vi "Format CSV.vi"(8 "error in (no error)":errorcluster, 9 "delimiter":string=",", 10 "CSV File Input":path, 11 "Original CSV Format":enum16{"Format A", "Format B"}(ring)) -> (0 "error out":errorcluster, 1 "Parcel Length":i32[](array[numeric]), 2 "All Terminal Data":T1(array[cluster]))   [LabVIEW 2017] (continued)
  in  "Start Time Selection":u16(ring) items=["20:35.0", "20:35.0", "20:35.1", "20:35.1", "20:35.1", "20:35.2", "20:35.2", "20:35.2", "20:35.3", "20:35.3", "20:35.3", "20:35.4", "20:35.4", "20:35.4", "20:35.5", "20:35.5", "20:35.5", "20:35.6", "20:35.6", "20:35.6", "20:35.7", "20:35.7", "20:35.7", "20:35.8", "20:35.8", "20:35.8", "20:35.9", "20:35.9", "20:35.9", "20:36.0", "20:36.0", "20:36.0", "20:36.1", "20:36.1", "20:36.1", "20:36.2", "20:36.2", "20:36.2", "20:36.3", "20:36.3", "20:36.3", "20:36.4", "20:36.4", "20:36.4", "20:36.5", "20:36.5", "20:36.5", "20:36.6", "20:36.6", "20:36.6", "20:36.7", "20:36.7", "20:36.7", "20:36.8", "20:36.8", "20:36.8", "20:36.9", "20:36.9", "20:36.9", "20:37.0", "20:37.0", "20:37.0", "20:37.1", "20:37.1", "20:37.1", "20:37.2", "20:37.2", "20:37.2", "20:37.3", "20:37.3", "20:37.3", "20:37.4", "20:37.4", "20:37.4", "20:37.5", "20:37.5", "20:37.5", "20:37.6", "20:37.6", "20:37.6", "20:37.7", "20:37.7", "20:37.7", "20:37.8", "20:37.8", "20:37.8", "20:37.9", "20:37.9", "20:37.9", "20:38.0", "20:38.0", "20:38.0", "20:38.1", "20:38.1", "20:38.1", "20:38.2", "20:38.2", "20:38.2", "20:38.3", "20:38.3", "20:38.3", "20:38.4", "20:38.4", "20:38.4", "20:38.5", "20:38.5", "20:38.5", "20:38.6", "20:38.6", "20:38.6", "20:38.7", "20:38.7", "20:38.7", "20:38.8", "20:38.8", "20:38.8", "20:38.9", "20:38.9", "20:38.9", "20:39.0", "20:39.0", "20:39.0", "20:39.1", "20:39.1", "20:39.1", "20:39.2", "20:39.2", "20:39.2", "20:39.3", "20:39.3", "20:39.3", "20:39.4", "20:39.4", "20:39.4", "20:39.5", "20:39.5", "20:39.5", "20:39.6", "20:39.6", "20:39.6", "20:39.7", "20:39.7", "20:39.7", "20:39.8", "20:39.8", "20:39.8", "20:39.9", "20:39.9", "20:39.9", "20:40.0", "20:40.0", "20:40.0", "20:40.1", "20:40.1", "20:40.1", "20:40.2", "20:40.2", "20:40.2", "20:40.3", "20:40.3", "20:40.3", "20:40.4", "20:40.4", "20:40.4", "20:40.5", "20:40.5", "20:40.5", "20:40.6", "20:40.6", "20:40.6", "20:40.7", "20:40.7", "20:40.7", "20:40.8", "20:40.8", "20:40.8", "20:40.9", "20:40.9", "20:40.9", "20:41.0", "20:41.0", "20:41.0", "20:41.1", "20:41.1", "20:41.1", "20:41.2", "20:41.2", "20:41.2", "20:41.3", "20:41.3", "20:41.3", "20:41.4", "20:41.4", "20:41.4", "20:41.5", "20:41.5", "20:41.5", "20:41.6", "20:41.6", "20:41.6", "20:41.7", "20:41.7", "20:41.7", "20:41.8", "20:41.8", "20:41.8", "20:41.9", "20:41.9", "20:41.9", "20:42.0", "20:42.0", "20:42.0", "20:42.1", "20:42.1", "20:42.1", "20:42.2", "20:42.2", "20:42.2", "20:42.3", "20:42.3", "20:42.3", "20:42.4", "20:42.4", "20:42.4", "20:42.5", "20:42.5", "20:42.5", "20:42.6", "20:42.6", "20:42.6", "20:42.7", "20:42.7", "20:42.7", "20:42.8", "20:42.8", "20:42.8", "20:42.9", "20:42.9", "20:42.9", "20:43.0", "20:43.0", "20:43.0", "20:43.1", "20:43.1", "20:43.1", "20:43.2", "20:43.2", "20:43.2", "20:43.3", "20:43.3", "20:43.3", "20:43.4", "20:43.4", "20:43.4", "20:43.5", "20:43.5", "20:43.5", "20:43.6", "20:43.6", "20:43.6", "20:43.7", "20:43.7", "20:43.7", "20:43.8", "20:43.8", "20:43.8", "20:43.9", "20:43.9", "20:43.9", "20:44.0", "20:44.0", "20:44.0", "20:44.1", "20:44.1", "20:44.1", "20:44.2", "20:44.2", "20:44.2", "20:44.3", "20:44.3", "20:44.3", "20:44.4", "20:44.4", "20:44.4", "20:44.5", "20:44.5", "20:44.5", "20:44.6", "20:44.6", "20:44.6", "20:44.7", "20:44.7", "20:44.7", "20:44.8", "20:44.8", "20:44.8", "20:44.9", "20:44.9", "20:44.9", "20:45.0", "20:45.0", "20:45.0", "20:45.1", "20:45.1", "20:45.1", "20:45.2", "20:45.2", "20:45.2", "20:45.3", "20:45.3", "20:45.3", "20:45.4", "20:45.4", "20:45.4", "20:45.5", "20:45.5", "20:45.5", "20:45.6", "20:45.6", "20:45.6", "20:45.7", "20:45.7", "20:45.7", "20:45.8", "20:45.8", "20:45.8", "20:45.9", "20:45.9", "20:45.9", "20:46.0", "20:46.0", "20:46.0", "20:46.1", "20:46.1", "20:46.1", "20:46.2", "20:46.2", "20:46.2", "20:46.3", "20:46.3", "20:46.3", "20:46.4", "20:46.4", "20:46.4", "20:46.5", "20:46.5", "20:46.5", "20:46.6", "20:46.6", "20:46.6", "20:46.7", "20:46.7", "20:46.7", "20:46.8", "20:46.8", "20:46.8", "20:46.9", "20:46.9", "20:46.9", "20:47.0", "20:47.0", "20:47.0", "20:47.1", "20:47.1", "20:47.1", "20:47.2", "20:47.2", "20:47.2", "20:47.3", "20:47.3", "20:47.3", "20:47.4", "20:47.4", "20:47.4", "20:47.5", "20:47.5", "20:47.5", "20:47.6", "20:47.6", "20:47.6", "20:47.7", "20:47.7", "20:47.7", "20:47.8", "20:47.8", "20:47.8", "20:47.9", "20:47.9", "20:47.9", "20:48.0", "20:48.0", "20:48.0", "20:48.1", "20:48.1", "20:48.1", "20:48.2", "20:48.2", "20:48.2", "20:48.3", "20:48.3", "20:48.3", "20:48.4", "20:48.4", "20:48.4", "20:48.5", "20:48.5", "20:48.5", "20:48.6", "20:48.6", "20:48.6", "20:48.7", "20:48.7", "20:48.7", "20:48.8", "20:48.8", "20:48.8", "20:48.9", "20:48.9", "20:48.9", "20:49.0", "20:49.0", "20:49.0", "20:49.1", "20:49.1", "20:49.1", "20:49.2", "20:49.2", "20:49.2", "20:49.3", "20:49.3", "20:49.3", "20:49.4", "20:49.4", "20:49.4", "20:49.5", "20:49.5", "20:49.5", "20:49.6", "20:49.6", "20:49.6", "20:49.7", "20:49.7", "20:49.7", "20:49.8", "20:49.8", "20:49.8", "20:49.9", "20:49.9", "20:49.9", "20:50.0", "20:50.0", "20:50.0", "20:50.1", "20:50.1", "20:50.1", "20:50.2", "20:50.2", "20:50.2", "20:50.3", "20:50.3", "20:50.3", "20:50.4", "20:50.4", "20:50.4", "20:50.5", "20:50.5", "20:50.5", "20:50.6", "20:50.6", "20:50.6", "20:50.7", "20:50.7", "20:50.7", "20:50.8", "20:50.8", "20:50.8", "20:50.9", "20:50.9", "20:50.9", "20:51.0", "20:51.0", "20:51.0", "20:51.1", "20:51.1", "20:51.1", "20:51.2", "20:51.2", "20:51.2", "20:51.3", "20:51.3", "20:51.3", "20:51.4", "20:51.4", "20:51.4", "20:51.5", "20:51.5", "20:51.5", "20:51.6", "20:51.6", "20:51.6", "20:51.7", "20:51.7", "20:51.7", "20:51.8", "20:51.8", "20:51.8", "20:51.9", "20:51.9", "20:51.9", "20:52.0", "20:52.0", "20:52.0", "20:52.1", "20:52.1", "20:52.1", "20:52.2", "20:52.2", "20:52.2", "20:52.3", "20:52.3", "20:52.3", "20:52.4", "20:52.4", "20:52.4", "20:52.5", "20:52.5", "20:52.5", "20:52.6", "20:52.6", "20:52.6", "20:52.7", "20:52.7", "20:52.7", "20:52.8", "20:52.8", "20:52.8", "20:52.9", "20:52.9", "20:52.9", "20:53.0", "20:53.0", "20:53.0", "20:53.1", "20:53.1", "20:53.1", "20:53.2", "20:53.2", "20:53.2", "20:53.3", "20:53.3", "20:53.3", "20:53.4", "20:53.4", "20:53.4", "20:53.5", "20:53.5", "20:53.5", "20:53.6", "20:53.6", "20:53.6", "20:53.7", "20:53.7", "20:53.7", "20:53.8", "20:53.8", "20:53.8", "20:53.9", "20:53.9", "20:53.9", "20:54.0", "20:54.0", "20:54.0", "20:54.1", "20:54.1", "20:54.1", "20:54.2", "20:54.2", "20:54.2", "20:54.3", "20:54.3", "20:54.3", "20:54.4", "20:54.4", "20:54.4", "20:54.5", "20:54.5", "20:54.5", "20:54.6", "20:54.6", "20:54.6", "20:54.7", "20:54.7", "20:54.7", "20:54.8", "20:54.8", "20:54.8", "20:54.9", "20:54.9", "20:54.9", "20:55.0", "20:55.0", "20:55.0", "20:55.1", "20:55.1", "20:55.1", "20:55.2", "20:55.2", "20:55.2", "20:55.3", "20:55.3", "20:55.3", "20:55.4", "20:55.4", "20:55.4", "20:55.5", "20:55.5", "20:55.5", "20:55.6", "20:55.6", "20:55.6", "20:55.7", "20:55.7", "20:55.7", "20:55.8", "20:55.8", "20:55.8", "20:55.9", "20:55.9", "20:55.9", "20:56.0", "20:56.0", "20:56.0", "20:56.1", "20:56.1", "20:56.1", "20:56.2", "20:56.2", "20:56.2", "20:56.3", "20:56.3", "20:56.3", "20:56.4", "20:56.4", "20:56.4", "20:56.5", "20:56.5", "20:56.5", "20:56.6", "20:56.6", "20:56.6", "20:56.7", "20:56.7", "20:56.7", "20:56.8", "20:56.8", "20:56.8", "20:56.9", "20:56.9", "20:56.9", "20:57.0", "20:57.0", "20:57.0", "20:57.1", "20:57.1", "20:57.1", "20:57.2", "20:57.2", "20:57.2", "20:57.3", "20:57.3", "20:57.3", "20:57.4", "20:57.4", "20:57.4", "20:57.5", "20:57.5", "20:57.5", "20:57.6", "20:57.6", "20:57.6", "20:57.7", "20:57.7", "20:57.7", "20:57.8", "20:57.8", "20:57.8", "20:57.9", "20:57.9", "20:57.9", "20:58.0", "20:58.0", "20:58.0", "20:58.1", "20:58.1", "20:58.1", "20:58.2", "20:58.2", "20:58.2", "20:58.3", "20:58.3", "20:58.3", "20:58.4", "20:58.4", "20:58.4", "20:58.5", "20:58.5", "20:58.5", "20:58.6", "20:58.6", "20:58.6", "20:58.7", "20:58.7", "20:58.7", "20:58.8", "20:58.8", "20:58.8", "20:58.9", "20:58.9", "20:58.9", "20:59.0", "20:59.0", "20:59.0", "20:59.1", "20:59.1", "20:59.1", "20:59.2", "20:59.2", "20:59.2", "20:59.3", "20:59.3", "20:59.3", "20:59.4", "20:59.4", "20:59.4", "20:59.5", "20:59.5", "20:59.5", "20:59.6", "20:59.6", "20:59.6", "20:59.7", "20:59.7", "20:59.7", "20:59.8", "20:59.8", "20:59.8", "20:59.9", "20:59.9", "20:59.9", "21:00.0", "21:00.0", "21:00.0", "21:00.1", "21:00.1", "21:00.1", "21:00.2", "21:00.2", "21:00.2", "21:00.3", "21:00.3", "21:00.3", "21:00.4", "21:00.4", "21:00.4", "21:00.5", "21:00.5", "21:00.5", "21:00.6", "21:00.6", "21:00.6", "21:00.7", "21:00.7", "21:00.7", "21:00.8", "21:00.8", "21:00.8", "21:00.9", "21:00.9", "21:00.9", "21:01.0", "21:01.0", "21:01.0", "21:01.1", "21:01.1", "21:01.1", "21:01.2", "21:01.2", "21:01.2", "21:01.3", "21:01.3", "21:01.3", "21:01.4", "21:01.4", "21:01.4", "21:01.5", "21:01.5", "21:01.5", "21:01.6", "21:01.6", "21:01.6", "21:01.7", "21:01.7", "21:01.7", "21:01.8", "21:01.8", "21:01.8", "21:01.9", "21:01.9", "21:01.9", "21:02.0", "21:02.0", "21:02.0", "21:02.1", "21:02.1", "21:02.1", "21:02.2", "21:02.2", "21:02.2", "21:02.3", "21:02.3", "21:02.3", "21:02.4", "21:02.4", "21:02.4", "21:02.5", "21:02.5", "21:02.5", "21:02.6", "21:02.6", "21:02.6", "21:02.7", "21:02.7", "21:02.7", "21:02.8", "21:02.8", "21:02.8", "21:02.9", "21:02.9", "21:02.9", "21:03.0", "21:03.0", "21:03.0", "21:03.1", "21:03.1", "21:03.1", "21:03.2", "21:03.2", "21:03.2", "21:03.3", "21:03.3", "21:03.3", "21:03.4", "21:03.4", "21:03.4", "21:03.5", "21:03.5", "21:03.5", "21:03.6", "21:03.6", "21:03.6", "21:03.7", "21:03.7", "21:03.7", "21:03.8", "21:03.8", "21:03.8", "21:03.9", "21:03.9", "21:03.9", "21:04.0", "21:04.0", "21:04.0", "21:04.1", "21:04.1", "21:04.1", "21:04.2", "21:04.2", "21:04.2", "21:04.3", "21:04.3", "21:04.3", "21:04.4", "21:04.4", "21:04.4", "21:04.5", "21:04.5", "21:04.5", "21:04.6", "21:04.6", "21:04.6", "21:04.7", "21:04.7", "21:04.7", "21:04.8", "21:04.8", "21:04.8", "21:04.9", "21:04.9", "21:04.9", "21:05.0", "21:05.0", "21:05.0", "21:05.1", "21:05.1", "21:05.1", "21:05.2", "21:05.2", "21:05.2", "21:05.3", "21:05.3", "21:05.3", "21:05.4", "21:05.4", "21:05.4", "21:05.5", "21:05.5", "21:05.5", "21:05.6", "21:05.6", "21:05.6", "21:05.7", "21:05.7", "21:05.7", "21:05.8", "21:05.8", "21:05.8", "21:05.9", "21:05.9", "21:05.9", "21:06.0", "21:06.0", "21:06.0", "21:06.1", "21:06.1", "21:06.1", "21:06.2", "21:06.2", "21:06.2", "21:06.3", "21:06.3", "21:06.3", "21:06.4", "21:06.4", "21:06.4", "21:06.5", "21:06.5", "21:06.5", "21:06.6", "21:06.6", "21:06.6", "21:06.7", "21:06.7", "21:06.7", "21:06.8", "21:06.8", "21:06.8", "21:06.9", "21:06.9", "21:06.9", "21:07.0", "21:07.0", "21:07.0", "21:07.1", "21:07.1", "21:07.1", "21:07.2", "21:07.2", "21:07.2", "21:07.3", "21:07.3", "21:07.3", "21:07.4", "21:07.4", "21:07.4", "21:07.5", "21:07.5", "21:07.5", "21:07.6", "21:07.6", "21:07.6", "21:07.7", "21:07.7", "21:07.7", "21:07.8", "21:07.8", "21:07.8", "21:07.9", "21:07.9", "21:07.9", "21:08.0", "21:08.0", "21:08.0", "21:08.1", "21:08.1", "21:08.1", "21:08.2", "21:08.2", "21:08.2", "21:08.3", "21:08.3", "21:08.3", "21:08.4", "21:08.4", "21:08.4", "21:08.5", "21:08.5", "21:08.5", "21:08.6", "21:08.6", "21:08.6", "21:08.7", "21:08.7", "21:08.7", "21:08.8", "21:08.8", "21:08.8", "21:08.9", "21:08.9", "21:08.9", "21:09.0", "21:09.0", "21:09.0", "21:09.1", "21:09.1", "21:09.1", "21:09.2", "21:09.2", "21:09.2", "21:09.3", "21:09.3", "21:09.3", "21:09.4", "21:09.4", "21:09.4", "21:09.5", "21:09.5", "21:09.5", "21:09.6", "21:09.6", "21:09.6", "21:09.7", "21:09.7", "21:09.7", "21:09.8", "21:09.8", "21:09.8", "21:09.9", "21:09.9", "21:09.9", "21:10.0", "21:10.0", "21:10.0", "21:10.1", "21:10.1", "21:10.1", "21:10.2", "21:10.2", "21:10.2", "21:10.3", "21:10.3", "21:10.3", "21:10.4", "21:10.4", "21:10.4", "21:10.5", "21:10.5", "21:10.5", "21:10.6", "21:10.6", "21:10.6", "21:10.7", "21:10.7", "21:10.7", "21:10.8", "21:10.8", "21:10.8", "21:10.9", "21:10.9", "21:10.9", "21:11.0", "21:11.0", "21:11.0", "21:11.1", "21:11.1", "21:11.1", "21:11.2", "21:11.2", "21:11.2", "21:11.3", "21:11.3", "21:11.3", "21:11.4", "21:11.4", "21:11.4", "21:11.5", "21:11.5", "21:11.5", "21:11.6", "21:11.6", "21:11.6", "21:11.7", "21:11.7", "21:11.7", "21:11.8", "21:11.8", "21:11.8", "21:11.9", "21:11.9", "21:11.9", "21:12.0", "21:12.0", "21:12.0", "21:12.1", "21:12.1", "21:12.1", "21:12.2", "21:12.2", "21:12.2", "21:12.3", "21:12.3", "21:12.3", "21:12.4", "21:12.4", "21:12.4", "21:12.5", "21:12.5", "21:12.5", "21:12.6", "21:12.6", "21:12.6", "21:12.7", "21:12.7", "21:12.7", "21:12.8", "21:12.8", "21:12.8", "21:12.9", "21:12.9", "21:12.9", "21:13.0", "21:13.0", "21:13.0", "21:13.1", "21:13.1", "21:13.1", "21:13.2", "21:13.2", "21:13.2", "21:13.3", "21:13.3", "21:13.3", "21:13.4", "21:13.4", "21:13.4", "21:13.5", "21:13.5", "21:13.5", "21:13.6", "21:13.6", "21:13.6", "21:13.7", "21:13.7", "21:13.7", "21:13.8", "21:13.8", "21:13.8", "21:13.9", "21:13.9", "21:13.9", "21:14.0", "21:14.0", "21:14.0", "21:14.1", "21:14.1", "21:14.1", "21:14.2", "21:14.2", "21:14.2", "21:14.3", "21:14.3", "21:14.3", "21:14.4", "21:14.4", "21:14.4", "21:14.5", "21:14.5", "21:14.5", "21:14.6", "21:14.6", "21:14.6", "21:14.7", "21:14.7", "21:14.7", "21:14.8", "21:14.8", "21:14.8", "21:14.9", "21:14.9", "21:14.9", "21:15.0", "21:15.0", "21:15.0", "21:15.1", "21:15.1", "21:15.1", "21:15.2", "21:15.2", "21:15.2", "21:15.3", "21:15.3", "21:15.3", "21:15.4", "21:15.4", "21:15.4", "21:15.5", "21:15.5", "21:15.5", "21:15.6", "21:15.6", "21:15.6", "21:15.7", "21:15.7", "21:15.7", "21:15.8", "21:15.8", "21:15.8", "21:15.9", "21:15.9", "21:15.9", "21:16.0", "21:16.0", "21:16.0", "21:16.1", "21:16.1", "21:16.1", "21:16.2", "21:16.2", "21:16.2", "21:16.3", "21:16.3", "21:16.3", "21:16.4", "21:16.4", "21:16.4", "21:16.5", "21:16.5", "21:16.5", "21:16.6", "21:16.6", "21:16.6", "21:16.7", "21:16.7", "21:16.7", "21:16.8", "21:16.8", "21:16.8", "21:16.9", "21:16.9", "21:16.9", "21:17.0", "21:17.0", "21:17.0", "21:17.1", "21:17.1", "21:17.1", "21:17.2", "21:17.2", "21:17.2", "21:17.3", "21:17.3", "21:17.3", "21:17.4", "21:17.4", "21:17.4", "21:17.5", "21:17.5", "21:17.5", "21:17.6", "21:17.6", "21:17.6", "21:17.7", "21:17.7", "21:17.7", "21:17.8", "21:17.8", "21:17.8", "21:17.9", "21:17.9", "21:17.9", "21:18.0", "21:18.0", "21:18.0", "21:18.1", "21:18.1", "21:18.1", "21:18.2", "21:18.2", "21:18.2", "21:18.3", "21:18.3", "21:18.3", "21:18.4", "21:18.4", "21:18.4", "21:18.5", "21:18.5", "21:18.5", "21:18.6", "21:18.6", "21:18.6", "21:18.7", "21:18.7", "21:18.7", "21:18.8", "21:18.8", "21:18.8", "21:18.9", "21:18.9", "21:18.9", "21:19.0", "21:19.0", "21:19.0", "21:19.1", "21:19.1", "21:19.1", "21:19.2", "21:19.2", "21:19.2", "21:19.3", "21:19.3", "21:19.3", "21:19.4", "21:19.4", "21:19.4", "21:19.5", "21:19.5", "21:19.5", "21:19.6", "21:19.6", "21:19.6", "21:19.7", "21:19.7", "21:19.7", "21:19.8", "21:19.8", "21:19.8", "21:19.9", "21:19.9", "21:19.9", "21:20.0", "21:20.0", "21:20.0", "21:20.1", "21:20.1", "21:20.1", "21:20.2", "21:20.2", "21:20.2", "21:20.3", "21:20.3", "21:20.3", "21:20.4", "21:20.4", "21:20.4", "21:20.5", "21:20.5", "21:20.5", "21:20.6", "21:20.6", "21:20.6", "21:20.7", "21:20.7", "21:20.7", "21:20.8", "21:20.8", "21:20.8", "21:20.9", "21:20.9", "21:20.9", "21:21.0", "21:21.0", "21:21.0", "21:21.1", "21:21.1", "21:21.1", "21:21.2", "21:21.2", "21:21.2", "21:21.3", "21:21.3", "21:21.3", "21:21.4", "21:21.4", "21:21.4", "21:21.5", "21:21.5", "21:21.5", "21:21.6", "21:21.6", "21:21.6", "21:21.7", "21:21.7", "21:21.7", "21:21.8", "21:21.8", "21:21.8", "21:21.9", "21:21.9", "21:21.9", "21:22.0", "21:22.0", "21:22.0", "21:22.1", "21:22.1", "21:22.1", "21:22.2", "21:22.2", "21:22.2", "21:22.3", "21:22.3", "21:22.3", "21:22.4", "21:22.4", "21:22.4", "21:22.5", "21:22.5", "21:22.5", "21:22.6", "21:22.6", "21:22.6", "21:22.7", "21:22.7", "21:22.7", "21:22.8", "21:22.8", "21:22.8", "21:22.9", "21:22.9", "21:22.9", "21:23.0", "21:23.0", "21:23.0", "21:23.1", "21:23.1", "21:23.1", "21:23.2", "21:23.2", "21:23.2", "21:23.3", "21:23.3", "21:23.3", "21:23.4", "21:23.4", "21:23.4", "21:23.5", "21:23.5", "21:23.5", "21:23.6", "21:23.6", "21:23.6", "21:23.7", "21:23.7", "21:23.7", "21:23.8", "21:23.8", "21:23.8", "21:23.9", "21:23.9", "21:23.9", "21:24.0", "21:24.0", "21:24.0", "21:24.1", "21:24.1", "21:24.1", "21:24.2", "21:24.2", "21:24.2", "21:24.3", "21:24.3", "21:24.3", "21:24.4", "21:24.4", "21:24.4", "21:24.5", "21:24.5", "21:24.5", "21:24.6", "21:24.6", "21:24.6", "21:24.7", "21:24.7", "21:24.7", "21:24.8", "21:24.8", "21:24.8", "21:24.9", "21:24.9", "21:24.9", "21:25.0", "21:25.0", "21:25.0", "21:25.1", "21:25.1", "21:25.1", "21:25.2", "21:25.2", "21:25.2", "21:25.3", "21:25.3", "21:25.3", "21:25.4", "21:25.4", "21:25.4", "21:25.5", "21:25.5", "21:25.5", "21:25.6", "21:25.6", "21:25.6", "21:25.7", "21:25.7", "21:25.7", "21:25.8", "21:25.8", "21:25.8", "21:25.9", "21:25.9", "21:25.9", "21:26.0", "21:26.0", "21:26.0", "21:26.1", "21:26.1", "21:26.1", "21:26.2", "21:26.2", "21:26.2", "21:26.3", "21:26.3", "21:26.3", "21:26.4", "21:26.4", "21:26.4", "21:26.5", "21:26.5", "21:26.5", "21:26.6", "21:26.6", "21:26.6", "21:26.7", "21:26.7", "21:26.7", "21:26.8", "21:26.8", "21:26.8", "21:26.9", "21:26.9", "21:26.9", "21:27.0", "21:27.0", "21:27.0", "21:27.1", "21:27.1", "21:27.1", "21:27.2", "21:27.2", "21:27.2", "21:27.3", "21:27.3", "21:27.3", "21:27.4", "21:27.4", "21:27.4", "21:27.5", "21:27.5", "21:27.5", "21:27.6", "21:27.6", "21:27.6", "21:27.7", "21:27.7", "21:27.7", "21:27.8", "21:27.8", "21:27.8", "21:27.9", "21:27.9", "21:27.9", "21:28.0", "21:28.0", "21:28.0", "21:28.1", "21:28.1", "21:28.1", "21:28.2", "21:28.2", "21:28.2", "21:28.3", "21:28.3", "21:28.3", "21:28.4", "21:28.4", "21:28.4", "21:28.5", "21:28.5", "21:28.5", "21:28.6", "21:28.6", "21:28.6", "21:28.7", "21:28.7", "21:28.7", "21:28.8", "21:28.8", "21:28.8", "21:28.9", "21:28.9", "21:28.9", "21:29.0", "21:29.0", "21:29.0", "21:29.1", "21:29.1", "21:29.1", "21:29.2", "21:29.2", "21:29.2", "21:29.3", "21:29.3", "21:29.3", "21:29.4", "21:29.4", "21:29.4", "21:29.5", "21:29.5", "21:29.5", "21:29.6", "21:29.6", "21:29.6", "21:29.7", "21:29.7", "21:29.7", "21:29.8", "21:29.8", "21:29.8", "21:29.9", "21:29.9", "21:29.9", "21:30.0", "21:30.0", "21:30.0", "21:30.1", "21:30.1", "21:30.1", "21:30.2", "21:30.2", "21:30.2", "21:30.3", "21:30.3", "21:30.3", "21:30.4", "21:30.4", "21:30.4", "21:30.5", "21:30.5", "21:30.5", "21:30.6", "21:30.6", "21:30.6", "21:30.7", "21:30.7", "21:30.7", "21:30.8", "21:30.8", "21:30.8", "21:30.9", "21:30.9", "21:30.9", "21:31.0", "21:31.0", "21:31.0", "21:31.1", "21:31.1", "21:31.1", "21:31.2", "21:31.2", "21:31.2", "21:31.3", "21:31.3", "21:31.3", "21:31.4", "21:31.4", "21:31.4", "21:31.5", "21:31.5", "21:31.5", "21:31.6", "21:31.6", "21:31.6", "21:31.7", "21:31.7", "21:31.7", "21:31.8", "21:31.8", "21:31.8", "21:31.9", "21:31.9", "21:31.9", "21:32.0", "21:32.0", "21:32.0", "21:32.1", "21:32.1", "21:32.1", "21:32.2", "21:32.2", "21:32.2", "21:32.3", "21:32.3", "21:32.3", "21:32.4", "21:32.4", "21:32.4", "21:32.5", "21:32.5", "21:32.5", "21:32.6", "21:32.6", "21:32.6", "21:32.7", "21:32.7", "21:32.7", "21:32.8", "21:32.8", "21:32.8", "21:32.9", "21:32.9", "21:32.9", "21:33.0", "21:33.0", "21:33.0", "21:33.1", "21:33.1", "21:33.1", "21:33.2", "21:33.2", "21:33.2", "21:33.3", "21:33.3", "21:33.3", "21:33.4", "21:33.4", "21:33.4", "21:33.5", "21:33.5", "21:33.5", "21:33.6", "21:33.6", "21:33.6", "21:33.7", "21:33.7", "21:33.7", "21:33.8", "21:33.8", "21:33.8", "21:33.9", "21:33.9", "21:33.9", "21:34.0", "21:34.0", "21:34.0", "21:34.1", "21:34.1", "21:34.1", "21:34.2", "21:34.2", "21:34.2", "21:34.3", "21:34.3", "21:34.3", "21:34.4", "21:34.4", "21:34.4", "21:34.5", "21:34.5", "21:34.5", "21:34.6", "21:34.6", "21:34.6", "21:34.7", "21:34.7", "21:34.7", "21:34.8", "21:34.8", "21:34.8", "21:34.9", "21:34.9", "21:34.9", "21:35.0", "21:35.0", "21:35.0", "21:35.1", "21:35.1", "21:35.1", "21:35.2", "21:35.2", "21:35.2", "21:35.3", "21:35.3", "21:35.3", "21:35.4", "21:35.4", "21:35.4", "21:35.5", "21:35.5", "21:35.5", "21:35.6", "21:35.6", "21:35.6", "21:35.7", "21:35.7", "21:35.7", "21:35.8", "21:35.8", "21:35.8", "21:35.9", "21:35.9", "21:35.9", "21:36.0", "21:36.0", "21:36.0", "21:36.1", "21:36.1", "21:36.1", "21:36.2", "21:36.2", "21:36.2", "21:36.3", "21:36.3", "21:36.3", "21:36.4", "21:36.4", "21:36.4", "21:36.5", "21:36.5", "21:36.5", "21:36.6", "21:36.6", "21:36.6", "21:36.7", "21:36.7", "21:36.7", "21:36.8", "21:36.8", "21:36.8", "21:36.9", "21:36.9", "21:36.9", "21:37.0", "21:37.0", "21:37.0", "21:37.1", "21:37.1", "21:37.1", "21:37.2", "21:37.2", "21:37.2", "21:37.3", "21:37.3", "21:37.3", "21:37.4", "21:37.4", "21:37.4", "21:37.5", "21:37.5", "21:37.5", "21:37.6", "21:37.6", "21:37.6", "21:37.7", "21:37.7", "21:37.7", "21:37.8", "21:37.8", "21:37.8", "21:37.9", "21:37.9", "21:37.9", "21:38.0", "21:38.0", "21:38.0", "21:38.1", "21:38.1", "21:38.1", "21:38.2", "21:38.2", "21:38.2", "21:38.3", "21:38.3", "21:38.3", "21:38.4", "21:38.4", "21:38.4", "21:38.5", "21:38.5", "21:38.5", "21:38.6", "21:38.6", "21:38.6", "21:38.7", "21:38.7", "21:38.7", "21:38.8", "21:38.8", "21:38.8", "21:38.9", "21:38.9", "21:38.9", "21:39.0", "21:39.0", "21:39.0", "21:39.1", "21:39.1", "21:39.1", "21:39.2", "21:39.2", "21:39.2", "21:39.3", "21:39.3", "21:39.3", "21:39.4", "21:39.4", "21:39.4", "21:39.5", "21:39.5", "21:39.5", "21:39.6", "21:39.6", "21:39.6", "21:39.7", "21:39.7", "21:39.7", "21:39.8", "21:39.8", "21:39.8", "21:39.9", "21:39.9", "21:39.9", "21:40.0", "21:40.0", "21:40.0", "21:40.1", "21:40.1", "21:40.1", "21:40.2", "21:40.2", "21:40.2", "21:40.3", "21:40.3", "21:40.3", "21:40.4", "21:40.4", "21:40.4", "21:40.5", "21:40.5", "21:40.5", "21:40.6", "21:40.6", "21:40.6", "21:40.7", "21:40.7", "21:40.7", "21:40.8", "21:40.8", "21:40.8", "21:40.9", "21:40.9", "21:40.9", "21:41.0", "21:41.0", "21:41.0", "21:41.1", "21:41.1", "21:41.1", "21:41.2", "21:41.2", "21:41.2", "21:41.3", "21:41.3", "21:41.3", "21:41.4", "21:41.4", "21:41.4", "21:41.5", "21:41.5", "21:41.5", "21:41.6", "21:41.6", "21:41.6", "21:41.7", "21:41.7", "21:41.7", "21:41.8", "21:41.8", "21:41.8", "21:41.9", "21:41.9", "21:41.9", "21:42.0", "21:42.0", "21:42.0", "21:42.1", "21:42.1", "21:42.1", "21:42.2", "21:42.2", "21:42.2", "21:42.3", "21:42.3", "21:42.3", "21:42.4", "21:42.4", "21:42.4", "21:42.5", "21:42.5", "21:42.5", "21:42.6", "21:42.6", "21:42.6", "21:42.7", "21:42.7", "21:42.7", "21:42.8", "21:42.8", "21:42.8", "21:42.9", "21:42.9", "21:42.9", "21:43.0", "21:43.0", "21:43.0", "21:43.1", "21:43.1", "21:43.1", "21:43.2", "21:43.2", "21:43.2", "21:43.3", "21:43.3", "21:43.3", "21:43.4", "21:43.4", "21:43.4", "21:43.5", "21:43.5", "21:43.5", "21:43.6", "21:43.6", "21:43.6", "21:43.7", "21:43.7", "21:43.7", "21:43.8", "21:43.8", "21:43.8", "21:43.9", "21:43.9", "21:43.9", "21:44.0", "21:44.0", "21:44.0", "21:44.1", "21:44.1", "21:44.1", "21:44.2", "21:44.2", "21:44.2", "21:44.3", "21:44.3", "21:44.3", "21:44.4", "21:44.4", "21:44.4", "21:44.5", "21:44.5", "21:44.5", "21:44.6", "21:44.6", "21:44.6", "21:44.7", "21:44.7", "21:44.7", "21:44.8", "21:44.8", "21:44.8", "21:44.9", "21:44.9", "21:44.9", "21:45.0", "21:45.0", "21:45.0", "21:45.1", "21:45.1", "21:45.1", "21:45.2", "21:45.2", "21:45.2", "21:45.3", "21:45.3", "21:45.3", "21:45.4", "21:45.4", "21:45.4", "21:45.5", "21:45.5", "21:45.5", "21:45.6", "21:45.6", "21:45.6", "21:45.7", "21:45.7", "21:45.7", "21:45.8", "21:45.8", "21:45.8", "21:45.9", "21:45.9", "21:45.9", "21:46.0", "21:46.0", "21:46.0", "21:46.1", "21:46.1", "21:46.1", "21:46.2", "21:46.2", "21:46.2", "21:46.3", "21:46.3", "21:46.3", "21:46.4", "21:46.4", "21:46.4", "21:46.5", "21:46.5", "21:46.5", "21:46.6", "21:46.6", "21:46.6", "21:46.7", "21:46.7", "21:46.7", "21:46.8", "21:46.8", "21:46.8", "21:46.9", "21:46.9", "21:46.9", "21:47.0", "21:47.0", "21:47.0", "21:47.1", "21:47.1", "21:47.1", "21:47.2", "21:47.2", "21:47.2", "21:47.3", "21:47.3", "21:47.3", "21:47.4", "21:47.4", "21:47.4", "21:47.5", "21:47.5", "21:47.5", "21:47.6", "21:47.6", "21:47.6", "21:47.7", "21:47.7", "21:47.7", "21:47.8", "21:47.8", "21:47.8", "21:47.9", "21:47.9", "21:47.9", "21:48.0", "21:48.0", "21:48.0", "21:48.1", "21:48.1", "21:48.1", "21:48.2", "21:48.2", "21:48.2", "21:48.3", "21:48.3", "21:48.3", "21:48.4", "21:48.4", "21:48.4", "21:48.5", "21:48.5", "21:48.5", "21:48.6", "21:48.6", "21:48.6", "21:48.7", "21:48.7", "21:48.7", "21:48.8", "21:48.8", "21:48.8", "21:48.9", "21:48.9", "21:48.9", "21:49.0", "21:49.0", "21:49.0", "21:49.1", "21:49.1", "21:49.1", "21:49.2", "21:49.2", "21:49.2", "21:49.3", "21:49.3", "21:49.3", "21:49.4", "21:49.4", "21:49.4", "21:49.5", "21:49.5", "21:49.5", "21:49.6", "21:49.6", "21:49.6", "21:49.7", "21:49.7", "21:49.7", "21:49.8", "21:49.8", "21:49.8", "21:49.9", "21:49.9", "21:49.9", "21:50.0", "21:50.0", "21:50.0", "21:50.1", "21:50.1", "21:50.1", "21:50.2", "21:50.2", "21:50.2", "21:50.3", "21:50.3", "21:50.3", "21:50.4", "21:50.4", "21:50.4", "21:50.5", "21:50.5", "21:50.5", "21:50.6", "21:50.6", "21:50.6", "21:50.7", "21:50.7", "21:50.7", "21:50.8", "21:50.8", "21:50.8", "21:50.9", "21:50.9", "21:50.9", "21:51.0", "21:51.0", "21:51.0", "21:51.1", "21:51.1", "21:51.1", "21:51.2", "21:51.2", "21:51.2", "21:51.3", "21:51.3", "21:51.3", "21:51.4", "21:51.4", "21:51.4", "21:51.5", "21:51.5", "21:51.5", "21:51.6", "21:51.6", "21:51.6", "21:51.7", "21:51.7", "21:51.7", "21:51.8", "21:51.8", "21:51.8", "21:51.9", "21:51.9", "21:51.9", "21:52.0", "21:52.0", "21:52.0", "21:52.1", "21:52.1", "21:52.1", "21:52.2", "21:52.2", "21:52.2", "21:52.3", "21:52.3", "21:52.3", "21:52.4", "21:52.4", "21:52.4", "21:52.5", "21:52.5", "21:52.5", "21:52.6", "21:52.6", "21:52.6", "21:52.7", "21:52.7", "21:52.7", "21:52.8", "21:52.8", "21:52.8", "21:52.9", "21:52.9", "21:52.9", "21:53.0", "21:53.0", "21:53.0", "21:53.1", "21:53.1", "21:53.1", "21:53.2", "21:53.2", "21:53.2", "21:53.3", "21:53.3", "21:53.3", "21:53.4", "21:53.4", "21:53.4", "21:53.5", "21:53.5", "21:53.5", "21:53.6", "21:53.6", "21:53.6", "21:53.7", "21:53.7", "21:53.7", "21:53.8", "21:53.8", "21:53.8", "21:53.9", "21:53.9", "21:53.9", "21:54.0", "21:54.0", "21:54.0", "21:54.1", "21:54.1", "21:54.1", "21:54.2", "21:54.2", "21:54.2", "21:54.3", "21:54.3", "21:54.3", "21:54.4", "21:54.4", "21:54.4", "21:54.5", "21:54.5", "21:54.5", "21:54.6", "21:54.6", "21:54.6", "21:54.7", "21:54.7", "21:54.7", "21:54.8", "21:54.8", "21:54.8", "21:54.9", "21:54.9", "21:54.9", "21:55.0", "21:55.0", "21:55.0", "21:55.1", "21:55.1", "21:55.1", "21:55.2", "21:55.2", "21:55.2", "21:55.3", "21:55.3", "21:55.3", "21:55.4", "21:55.4", "21:55.4", "21:55.5", "21:55.5", "21:55.5", "21:55.6", "21:55.6", "21:55.6", "21:55.7", "21:55.7", "21:55.7", "21:55.8", "21:55.8", "21:55.8", "21:55.9", "21:55.9", "21:55.9", "21:56.0", "21:56.0", "21:56.0", "21:56.1", "21:56.1", "21:56.1", "21:56.2", "21:56.2", "21:56.2", "21:56.3", "21:56.3", "21:56.3", "21:56.4", "21:56.4", "21:56.4", "21:56.5", "21:56.5", "21:56.5", "21:56.6", "21:56.6", "21:56.6", "21:56.7", "21:56.7", "21:56.7", "21:56.8", "21:56.8", "21:56.8", "21:56.9", "21:56.9", "21:56.9", "21:57.0", "21:57.0", "21:57.0", "21:57.1", "21:57.1", "21:57.1", "21:57.2", "21:57.2", "21:57.2", "21:57.3", "21:57.3", "21:57.3", "21:57.4", "21:57.4", "21:57.4", "21:57.5", "21:57.5", "21:57.5", "21:57.6", "21:57.6", "21:57.6", "21:57.7", "21:57.7", "21:57.7", "21:57.8", "21:57.8", "21:57.8", "21:57.9", "21:57.9", "21:57.9", "21:58.0", "21:58.0", "21:58.0", "21:58.1", "21:58.1", "21:58.1", "21:58.2", "21:58.2", "21:58.2", "21:58.3", "21:58.3", "21:58.3", "21:58.4", "21:58.4", "21:58.4", "21:58.5", "21:58.5", "21:58.5", "21:58.6", "21:58.6", "21:58.6", "21:58.7", "21:58.7", "21:58.7", "21:58.8", "21:58.8", "21:58.8", "21:58.9", "21:58.9", "21:58.9", "21:59.0", "21:59.0", "21:59.0", "21:59.1", "21:59.1", "21:59.1", "21:59.2", "21:59.2", "21:59.2", "21:59.3", "21:59.3", "21:59.3", "21:59.4", "21:59.4", "21:59.4", "21:59.5", "21:59.5", "21:59.5", "21:59.6", "21:59.6", "21:59.6", "21:59.7", "21:59.7", "21:59.7", "21:59.8", "21:59.8", "21:59.8", "21:59.9", "21:59.9", "21:59.9", "22:00.0", "22:00.0", "22:00.0", "22:00.1", "22:00.1", "22:00.1", "22:00.2", "22:00.2", "22:00.2", "22:00.3", "22:00.3", "22:00.3", "22:00.4", "22:00.4", "22:00.4", "22:00.5", "22:00.5", "22:00.5", "22:00.6", "22:00.6", "22:00.6", "22:00.7", "22:00.7", "22:00.7", "22:00.8", "22:00.8", "22:00.8", "22:00.9", "22:00.9", "22:00.9", "22:01.0", "22:01.0", "22:01.0", "22:01.1", "22:01.1", "22:01.1", "22:01.2", "22:01.2", "22:01.2", "22:01.3", "22:01.3", "22:01.3", "22:01.4", "22:01.4", "22:01.4", "22:01.5", "22:01.5", "22:01.5", "22:01.6", "22:01.6", "22:01.6", "22:01.7", "22:01.7", "22:01.7", "22:01.8", "22:01.8", "22:01.8", "22:01.9", "22:01.9", "22:01.9", "22:02.0", "22:02.0", "22:02.0", "22:02.1", "22:02.1", "22:02.1", "22:02.2", "22:02.2", "22:02.2", "22:02.3", "22:02.3", "22:02.3", "22:02.4", "22:02.4", "22:02.4", "22:02.5", "22:02.5", "22:02.5", "22:02.6", "22:02.6", "22:02.6", "22:02.7", "22:02.7", "22:02.7", "22:02.8", "22:02.8", "22:02.8", "22:02.9", "22:02.9", "22:02.9", "22:03.0", "22:03.0", "22:03.0", "22:03.1", "22:03.1", "22:03.1", "22:03.2", "22:03.2", "22:03.2", "22:03.3", "22:03.3", "22:03.3", "22:03.4", "22:03.4", "22:03.4", "22:03.5", "22:03.5", "22:03.5", "22:03.6", "22:03.6", "22:03.6", "22:03.7", "22:03.7", "22:03.7", "22:03.8", "22:03.8", "22:03.8", "22:03.9", "22:03.9", "22:03.9", "22:04.0", "22:04.0", "22:04.0", "22:04.1", "22:04.1", "22:04.1", "22:04.2", "22:04.2", "22:04.2", "22:04.3", "22:04.3", "22:04.3", "22:04.4", "22:04.4", "22:04.4", "22:04.5", "22:04.5", "22:04.5", "22:04.6", "22:04.6", "22:04.6", "22:04.7", "22:04.7", "22:04.7", "22:04.8", "22:04.8", "22:04.8", "22:04.9", "22:04.9", "22:04.9", "22:05.0", "22:05.0", "22:05.0", "22:05.1", "22:05.1", "22:05.1", "22:05.2", "22:05.2", "22:05.2", "22:05.3", "22:05.3", "22:05.3", "22:05.4", "22:05.4", "22:05.4", "22:05.5", "22:05.5", "22:05.5", "22:05.6", "22:05.6", "22:05.6", "22:05.7", "22:05.7", "22:05.7", "22:05.8", "22:05.8", "22:05.8", "22:05.9", "22:05.9", "22:05.9", "22:06.0", "22:06.0", "22:06.0", "22:06.1", "22:06.1", "22:06.1", "22:06.2", "22:06.2", "22:06.2", "22:06.3", "22:06.3", "22:06.3", "22:06.4", "22:06.4", "22:06.4", "22:06.5", "22:06.5", "22:06.5", "22:06.6", "22:06.6", "22:06.6", "22:06.7", "22:06.7", "22:06.7", "22:06.8", "22:06.8", "22:06.8", "22:06.9", "22:06.9", "22:06.9", "22:07.0", "22:07.0", "22:07.0", "22:07.1", "22:07.1", "22:07.1", "22:07.2", "22:07.2", "22:07.2", "22:07.3", "22:07.3", "22:07.3", "22:07.4", "22:07.4", "22:07.4", "22:07.5", "22:07.5", "22:07.5", "22:07.6", "22:07.6", "22:07.6", "22:07.7", "22:07.7", "22:07.7", "22:07.8", "22:07.8", "22:07.8", "22:07.9", "22:07.9", "22:07.9", "22:08.0", "22:08.0", "22:08.0", "22:08.1", "22:08.1", "22:08.1", "22:08.2", "22:08.2", "22:08.2", "22:08.3", "22:08.3", "22:08.3", "22:08.4", "22:08.4", "22:08.4", "22:08.5", "22:08.5", "22:08.5", "22:08.6", "22:08.6", "22:08.6", "22:08.7", "22:08.7", "22:08.7", "22:08.8", "22:08.8", "22:08.8", "22:08.9", "22:08.9", "22:08.9", "22:09.0", "22:09.0", "22:09.0", "22:09.1", "22:09.1", "22:09.1", "22:09.2", "22:09.2", "22:09.2", "22:09.3", "22:09.3", "22:09.3", "22:09.4", "22:09.4", "22:09.4", "22:09.5", "22:09.5", "22:09.5", "22:09.6", "22:09.6", "22:09.6", "22:09.7", "22:09.7", "22:09.7", "22:09.8", "22:09.8", "22:09.8", "22:09.9", "22:09.9", "22:09.9", "22:10.0", "22:10.0", "22:10.0", "22:10.1", "22:10.1", "22:10.1", "22:10.2", "22:10.2", "22:10.2", "22:10.3", "22:10.3", "22:10.3", "22:10.4", "22:10.4", "22:10.4", "22:10.5", "22:10.5", "22:10.5", "22:10.6", "22:10.6", "22:10.6", "22:10.7", "22:10.7", "22:10.7", "22:10.8", "22:10.8", "22:10.8", "22:10.9", "22:10.9", "22:10.9", "22:11.0", "22:11.0", "22:11.0", "22:11.1", "22:11.1", "22:11.1", "22:11.2", "22:11.2", "22:11.2", "22:11.3", "22:11.3", "22:11.3", "22:11.4", "22:11.4", "22:11.4", "22:11.5", "22:11.5", "22:11.5", "22:11.6", "22:11.6", "22:11.6", "22:11.7", "22:11.7", "22:11.7", "22:11.8", "22:11.8", "22:11.8", "22:11.9", "22:11.9", "22:11.9", "22:12.0", "22:12.0", "22:12.0", "22:12.1", "22:12.1", "22:12.1", "22:12.2", "22:12.2", "22:12.2", "22:12.3", "22:12.3", "22:12.3", "22:12.4", "22:12.4", "22:12.4", "22:12.5", "22:12.5", "22:12.5", "22:12.6", "22:12.6", "22:12.6", "22:12.7", "22:12.7", "22:12.7", "22:12.8", "22:12.8", "22:12.8", "22:12.9", "22:12.9", "22:12.9", "22:13.0", "22:13.0", "22:13.0", "22:13.1", "22:13.1", "22:13.1", "22:13.2", "22:13.2", "22:13.2", "22:13.3", "22:13.3", "22:13.3", "22:13.4", "22:13.4", "22:13.4", "22:13.5", "22:13.5", "22:13.5", "22:13.6", "22:13.6", "22:13.6", "22:13.7", "22:13.7", "22:13.7", "22:13.8", "22:13.8", "22:13.8", "22:13.9", "22:13.9", "22:13.9", "22:14.0", "22:14.0", "22:14.0", "22:14.1", "22:14.1", "22:14.1", "22:14.2", "22:14.2", "22:14.2", "22:14.3", "22:14.3", "22:14.3", "22:14.4", "22:14.4", "22:14.4", "22:14.5", "22:14.5", "22:14.5", "22:14.6", "22:14.6", "22:14.6", "22:14.7", "22:14.7", "22:14.7", "22:14.8", "22:14.8", "22:14.8", "22:14.9", "22:14.9", "22:14.9", "22:15.0", "22:15.0", "22:15.0", "22:15.1", "22:15.1", "22:15.1", "22:15.2", "22:15.2", "22:15.2", "22:15.3", "22:15.3", "22:15.3", "22:15.4", "22:15.4", "22:15.4", "22:15.5", "22:15.5", "22:15.5", "22:15.6", "22:15.6", "22:15.6", "22:15.7", "22:15.7", "22:15.7", "22:15.8", "22:15.8", "22:15.8", "22:15.9", "22:15.9", "22:15.9", "22:16.0", "22:16.0", "22:16.0", "22:16.1", "22:16.1", "22:16.1", "22:16.2", "22:16.2", "22:16.2", "22:16.3", "22:16.3", "22:16.3", "22:16.4", "22:16.4", "22:16.4", "22:16.5", "22:16.5", "22:16.5", "22:16.6", "22:16.6", "22:16.6", "22:16.7", "22:16.7", "22:16.7", "22:16.8", "22:16.8", "22:16.8", "22:16.9", "22:16.9", "22:16.9", "22:17.0", "22:17.0", "22:17.0", "22:17.1", "22:17.1", "22:17.1", "22:17.2", "22:17.2", "22:17.2", "22:17.3", "22:17.3", "22:17.3", "22:17.4", "22:17.4", "22:17.4", "22:17.5", "22:17.5", "22:17.5", "22:17.6", "22:17.6", "22:17.6", "22:17.7", "22:17.7", "22:17.7", "22:17.8", "22:17.8", "22:17.8", "22:17.9", "22:17.9", "22:17.9", "22:18.0", "22:18.0", "22:18.0", "22:18.1", "22:18.1", "22:18.1", "22:18.2", "22:18.2", "22:18.2", "22:18.3", "22:18.3", "22:18.3", "22:18.4", "22:18.4", "22:18.4", "22:18.5", "22:18.5", "22:18.5", "22:18.6", "22:18.6", "22:18.6", "22:18.7", "22:18.7", "22:18.7", "22:18.8", "22:18.8", "22:18.8", "22:18.9", "22:18.9", "22:18.9", "22:19.0", "22:19.0", "22:19.0", "22:19.1", "22:19.1", "22:19.1", "22:19.2", "22:19.2", "22:19.2", "22:19.3", "22:19.3", "22:19.3", "22:19.4", "22:19.4", "22:19.4", "22:19.5", "22:19.5", "22:19.5", "22:19.6", "22:19.6", "22:19.6", "22:19.7", "22:19.7", "22:19.7", "22:19.8", "22:19.8", "22:19.8", "22:19.9", "22:19.9", "22:19.9", "22:20.0", "22:20.0", "22:20.0", "22:20.1", "22:20.1", "22:20.1", "22:20.2", "22:20.2", "22:20.2", "22:20.3", "22:20.3", "22:20.3", "22:20.4", "22:20.4", "22:20.4", "22:20.5", "22:20.5", "22:20.5", "22:20.6", "22:20.6", "22:20.6", "22:20.7", "22:20.7", "22:20.7", "22:20.8", "22:20.8", "22:20.8", "22:20.9", "22:20.9", "22:20.9", "22:21.0", "22:21.0", "22:21.0", "22:21.1", "22:21.1", "22:21.1", "22:21.2", "22:21.2", "22:21.2", "22:21.3", "22:21.3", "22:21.3", "22:21.4", "22:21.4", "22:21.4", "22:21.5", "22:21.5", "22:21.5", "22:21.6", "22:21.6", "22:21.6", "22:21.7", "22:21.7", "22:21.7", "22:21.8", "22:21.8", "22:21.8", "22:21.9", "22:21.9", "22:21.9", "22:22.0", "22:22.0", "22:22.0", "22:22.1", "22:22.1", "22:22.1", "22:22.2", "22:22.2", "22:22.2", "22:22.3", "22:22.3", "22:22.3", "22:22.4", "22:22.4", "22:22.4", "22:22.5", "22:22.5", "22:22.5", "22:22.6", "22:22.6", "22:22.6", "22:22.7", "22:22.7", "22:22.7", "22:22.8", "22:22.8", "22:22.8", "22:22.9", "22:22.9", "22:22.9", "22:23.0", "22:23.0", "22:23.0", "22:23.1", "22:23.1", "22:23.1", "22:23.2", "22:23.2", "22:23.2", "22:23.3", "22:23.3", "22:23.3", "22:23.4", "22:23.4", "22:23.4", "22:23.5", "22:23.5", "22:23.5", "22:23.6", "22:23.6", "22:23.6", "22:23.7", "22:23.7", "22:23.7", "22:23.8", "22:23.8", "22:23.8", "22:23.9", "22:23.9", "22:23.9", "22:24.0", "22:24.0", "22:24.0", "22:24.1", "22:24.1", "22:24.1", "22:24.2", "22:24.2", "22:24.2", "22:24.3", "22:24.3", "22:24.3", "22:24.4", "22:24.4", "22:24.4", "22:24.5", "22:24.5", "22:24.5", "22:24.6", "22:24.6", "22:24.6", "22:24.7", "22:24.7", "22:24.7", "22:24.8", "22:24.8", "22:24.8", "22:24.9", "22:24.9", "22:24.9", "22:25.0", "22:25.0", "22:25.0", "22:25.1", "22:25.1", "22:25.1", "22:25.2", "22:25.2", "22:25.2", "22:25.3", "22:25.3", "22:25.3", "22:25.4", "22:25.4", "22:25.4", "22:25.5", "22:25.5", "22:25.5", "22:25.6", "22:25.6", "22:25.6", "22:25.7", "22:25.7", "22:25.7", "22:25.8", "22:25.8", "22:25.8", "22:25.9", "22:25.9", "22:25.9", "22:26.0", "22:26.0", "22:26.0", "22:26.1", "22:26.1", "22:26.1", "22:26.2", "22:26.2", "22:26.2", "22:26.3", "22:26.3", "22:26.3", "22:26.4", "22:26.4", "22:26.4", "22:26.5", "22:26.5", "22:26.5", "22:26.6", "22:26.6", "22:26.6", "22:26.7", "22:26.7", "22:26.7", "22:26.8", "22:26.8", "22:26.8", "22:26.9", "22:26.9", "22:26.9", "22:27.0", "22:27.0", "22:27.0", "22:27.1", "22:27.1", "22:27.1", "22:27.2", "22:27.2", "22:27.2", "22:27.3", "22:27.3", "22:27.3", "22:27.4", "22:27.4", "22:27.4", "22:27.5", "22:27.5", "22:27.5", "22:27.6", "22:27.6", "22:27.6", "22:27.7", "22:27.7", "22:27.7", "22:27.8", "22:27.8", "22:27.8", "22:27.9", "22:27.9", "22:27.9", "22:28.0", "22:28.0", "22:28.0", "22:28.1", "22:28.1", "22:28.1", "22:28.2", "22:28.2", "22:28.2", "22:28.3", "22:28.3", "22:28.3", "22:28.4", "22:28.4", "22:28.4", "22:28.5", "22:28.5", "22:28.5", "22:28.6", "22:28.6", "22:28.6", "22:28.7", "22:28.7", "22:28.7", "22:28.8", "22:28.8", "22:28.8", "22:28.9", "22:28.9", "22:28.9", "22:29.0", "22:29.0", "22:29.0", "22:29.1", "22:29.1", "22:29.1", "22:29.2", "22:29.2", "22:29.2", "22:29.3", "22:29.3", "22:29.3", "22:29.4", "22:29.4", "22:29.4", "22:29.5", "22:29.5", "22:29.5", "22:29.6", "22:29.6", "22:29.6", "22:29.7", "22:29.7", "22:29.7", "22:29.8", "22:29.8", "22:29.8", "22:29.9", "22:29.9", "22:29.9", "22:30.0", "22:30.0", "22:30.0", "22:30.1", "22:30.1", "22:30.1", "22:30.2", "22:30.2", "22:30.2", "22:30.3", "22:30.3", "22:30.3", "22:30.4", "22:30.4", "22:30.4", "22:30.5", "22:30.5", "22:30.5", "22:30.6", "22:30.6", "22:30.6", "22:30.7", "22:30.7", "22:30.7", "22:30.8", "22:30.8", "22:30.8", "22:30.9", "22:30.9", "22:30.9", "22:31.0", "22:31.0", "22:31.0", "22:31.1", "22:31.1", "22:31.1", "22:31.2", "22:31.2", "22:31.2", "22:31.3", "22:31.3", "22:31.3", "22:31.4", "22:31.4", "22:31.4", "22:31.5", "22:31.5", "22:31.5", "22:31.6", "22:31.6", "22:31.6", "22:31.7", "22:31.7", "22:31.7", "22:31.8", "22:31.8", "22:31.8", "22:31.9", "22:31.9", "22:31.9", "22:32.0", "22:32.0", "22:32.0", "22:32.1", "22:32.1", "22:32.1", "22:32.2", "22:32.2", "22:32.2", "22:32.3", "22:32.3", "22:32.3", "22:32.4", "22:32.4", "22:32.4", "22:32.5", "22:32.5", "22:32.5", "22:32.6", "22:32.6", "22:32.6", "22:32.7", "22:32.7", "22:32.7", "22:32.8", "22:32.8", "22:32.8", "22:32.9", "22:32.9", "22:32.9", "22:33.0", "22:33.0", "22:33.0", "22:33.1", "22:33.1", "22:33.1", "22:33.2", "22:33.2", "22:33.2", "22:33.3", "22:33.3", "22:33.3", "22:33.4", "22:33.4", "22:33.4", "22:33.5", "22:33.5", "22:33.5", "22:33.6", "22:33.6", "22:33.6", "22:33.7", "22:33.7", "22:33.7", "22:33.8", "22:33.8", "22:33.8", "22:33.9", "22:33.9", "22:33.9", "22:34.0", "22:34.0", "22:34.0", "22:34.1", "22:34.1", "22:34.1", "22:34.2", "22:34.2", "22:34.2", "22:34.3", "22:34.3", "22:34.3", "22:34.4", "22:34.4", "22:34.4", "22:34.5", "22:34.5", "22:34.5", "22:34.6", "22:34.6", "22:34.6", "22:34.7", "22:34.7", "22:34.7", "22:34.8", "22:34.8", "22:34.8", "22:34.9", "22:34.9", "22:34.9", "22:35.0", "22:35.0", "22:35.0", "22:35.1", "22:35.1", "22:35.1", "22:35.2", "22:35.2", "22:35.2", "22:35.3", "22:35.3", "22:35.3", "22:35.4", "22:35.4", "22:35.4", "22:35.5", "22:35.5", "22:35.5", "22:35.6", "22:35.6", "22:35.6", "22:35.7", "22:35.7", "22:35.7", "22:35.8", "22:35.8", "22:35.8", "22:35.9", "22:35.9", "22:35.9", "22:36.0", "22:36.0", "22:36.0", "22:36.1", 
